vi "HVAC_Control_subTest.vi"(7 "Test Result in":T2=enum."Success", 8 "error in":errorcluster, 9 "DeviceID":T1, 10 "MicrogridID":u8, 11 "Message Enqueuer in":refnum<class "Message Enqueuer.lvclass">) -> (0 "error out":errorcluster, 1 "dup DeviceID":T1, 2 "dup MicrogridID":u8, 3 "Message Enqueuer out":refnum<class "Message Enqueuer.lvclass">, 5 "Test Result out":T2=enum."Success")   [LabVIEW 2018, in "IED Test Framework.lvlib" / "IED Test.lvclass"]
doc: "This VI tests Activate and Deactive messages as part of DER_Control."
uses:
  IED Test.lvclass
  Controls/Test Result.ctl
  <vilib>/ORNL/CSEISMIC DDS/CSEISMIC DDS Base/Data Types/Controls/DeviceID.ctl
  <vilib>/ActorFramework/Message Enqueuer/Message Enqueuer.lvclass
  <vilib>/ORNL/CSEISMIC DDS/CSEISMIC DDS Base/Data Types/Controls/ControlMode.ctl
  <vilib>/ORNL/CSEISMIC DDS/CSEISMIC DDS Base/Data Types/HVAC_Control.ctl
  <vilib>/ORNL/CSEISMIC DDS/CSEISMIC DDS Base/CSEISMIC DDS.lvclass/CSEISMIC DDS.ctl
  HVAC Actor/HVAC Messages/Write HVAC Control Msg/Write HVAC Control Msg.lvclass/Write HVAC Control Msg.ctl
  <vilib>/ActorFramework/Message Enqueuer/Message Enqueuer.lvclass/Message Enqueuer.ctl
  <vilib>/ORNL/CSEISMIC DDS/CSEISMIC DDS Base/Accessors/Write DDS Reference.vi
  <vilib>/ActorFramework/Message Enqueuer/Enqueue.vi
  <vilib>/ORNL/CSEISMIC DDS/CSEISMIC DDS Base/Accessors/Read DDS Reference.vi
  <vilib>/ORNL/CSEISMIC DDS/DDS Reader/DDS Reader.lvclass
  C:/Program Files (x86)/National Instruments/LabVIEW 2018/vi.lib/ORNL/CSEISMIC DDS/CSEISMIC DDS Base/CSEISMIC DDS.lvclass
  HVAC Actor/HVAC Messages/Write HVAC Control Msg/Write HVAC Control Msg.lvclass
  C:/Program Files (x86)/National Instruments/LabVIEW 2018/vi.lib/ActorFramework/Message/Message.lvclass
  <vilib>/ORNL/CSEISMIC DDS/CSEISMIC DDS Base/Error Handler.vi
  <vilib>/ActorFramework/Message Priority Queue/Priority Enqueue.vi
  <vilib>/ORNL/CSEISMIC DDS/CSEISMIC DDS Base/CSEISMIC DDS.lvclass
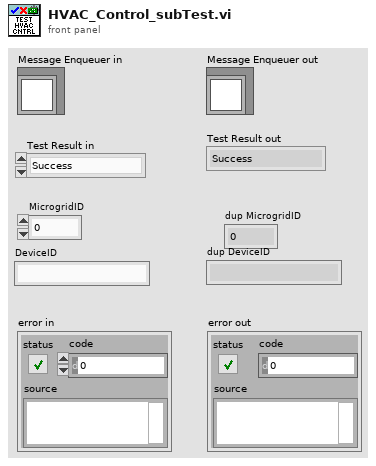
[diagram p1: front panel]
types:
  T1 = typedef "CSEISMIC DDS.lvlib/CSEISMIC DDS.lvclass/DeviceID.ctl" = string
  T2 = typedef "IED Test Framework.lvlib/IED Test.lvclass/Test Result.ctl" = enum16{"Invalid", "Success", "Failure", "Error", "Timeout"}
  T3 = typedef "CSEISMIC DDS.lvlib/CSEISMIC DDS.lvclass/ControlMode.ctl" = enum32{"Invalid", "Cooling", "Heating"}
  T4 = typedef "CSEISMIC DDS.lvlib/CSEISMIC DDS.lvclass/HVAC_Control.ctl" = cluster{"DeviceID":T1, "Temperature(degC)":dbl, "ControlMode":T3}
  T5 = typedef "LVDDS_library.lvlib/DDS Sample Info.ctl" = cluster{"DDS_SampleStateKind":enum32{"DDS_INVALID_SAMPLE_STATE", "DDS_READ_SAMPLE_STATE", "DDS_NOT_READ_SAMPLE_STATE"}, "DDS_ViewStateKind":enum32{"DDS_INVALID_SAMPLE_STATE", "DDS_NEW_VIEW_STATE", "DDS_NOT_NEW_VIEW_STATE"}, "DDS_InstanceStateKind":enum32{"DDS_INVALID_STATE", "DDS_ALIVE_INSTANCE_STATE", "DDS_NOT_ALIVE_DISPOSED_INSTANCE_STATE", "", "DDS_NOT_ALIVE_NO_WRITERS_INSTANCE_STATE"}, "sec":i32, "nanosec":u32, "valid_data":bool}
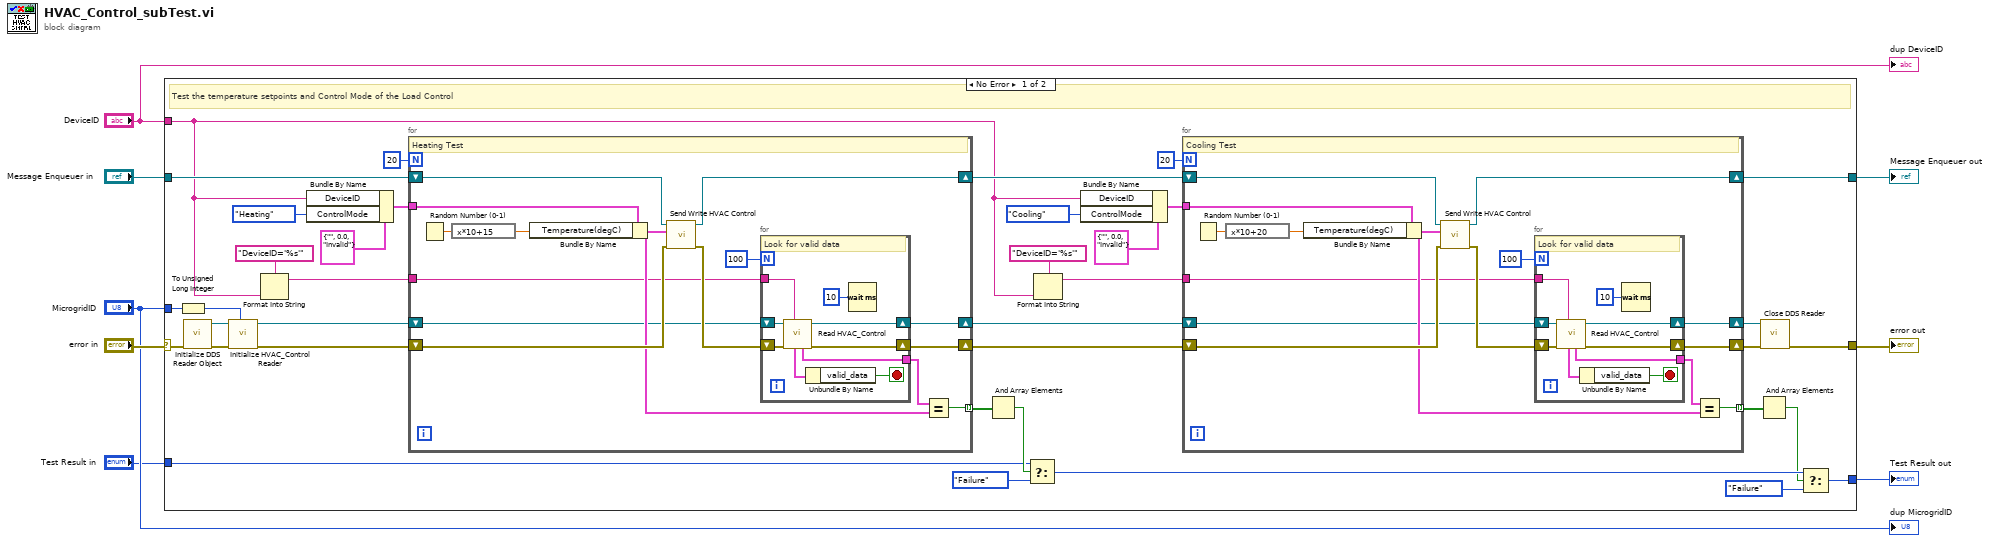
[diagram p0: block diagram]
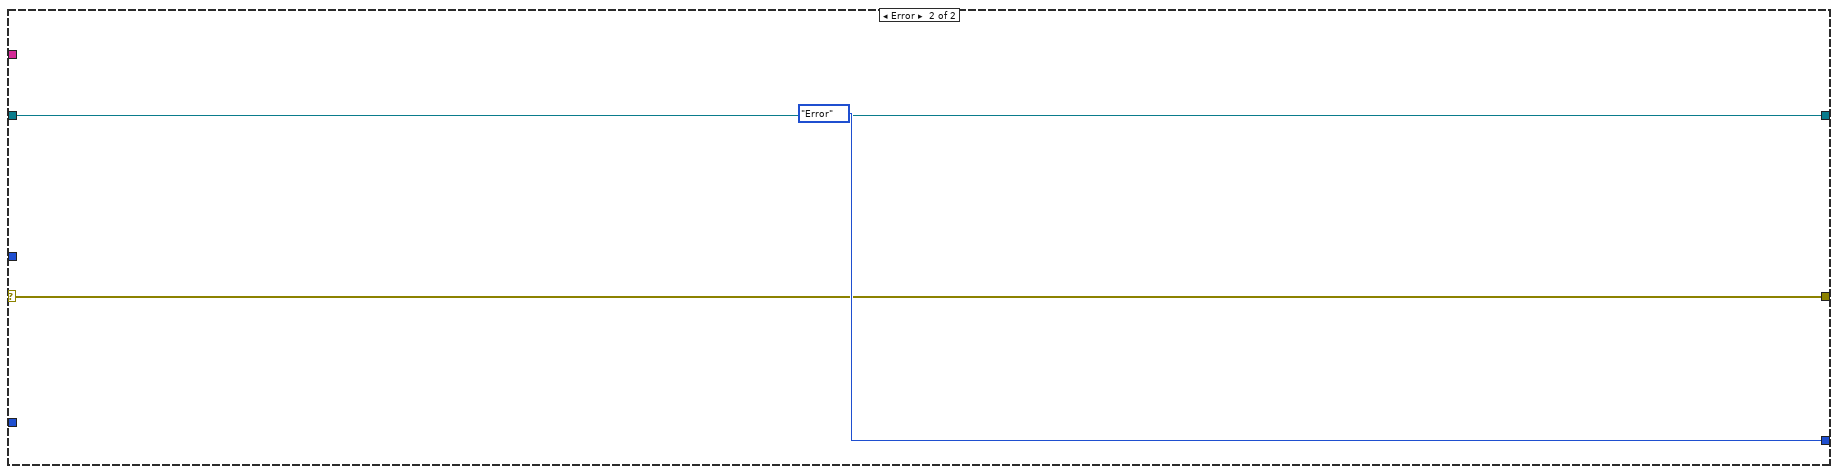
[diagram p2: hidden frame]
diagram:
  n1 = case shown="No Error" "error in" {
    selector: "error in" -> [w33 w95]
    tunnel: [w35 Test_Result."Error" ("Test Result")] -> w8
    tunnel: "DeviceID" -> [w14 _]
    tunnel: [w9 w94] -> w7
    tunnel: "MicrogridID" -> [w32 _]
    tunnel: [w10 w95] -> w6
    tunnel: "Message Enqueuer in" -> [w42 w94]
    tunnel: "Test Result in" -> [w38 _]
    frame No Error {
      # "Test the temperature setpoints and Control Mode of the Load Control"
      n2 = To Unsigned Long Integer(number=w32) -> (unsigned 32bit integer=w29:u32)
      n3 = call <vilib>:"Initialize DDS Reader Object.vi"("error in"=w33) -> ("error out"=w31:errorcluster, "DDS Reader out"=w30:refnum<class "DDS Reader.lvclass">)  [unwired: 9 in]
      n4 = call <vilib>:"Initialize HVAC_Control Reader.vi"("MicrogridID"=w29, "error in"=w31, "DDS Reader in"=w30) -> ("error out"=w28:errorcluster, "DDS Reader out"=w27:refnum<class "DDS Reader.lvclass">)  [unwired: 7 in]
      n5 = Format Into String(format string="DeviceID='%s'", w14) -> (resulting string=w25:string)  [unwired: 2 in, 1 out]
      n6 = Bundle By Name(cluster=T4 {"DeviceID"="", "Temperature(degC)"=0.0, "ControlMode"=enum."Invalid"} ("HVAC_Control"), "DeviceID"=w14, "ControlMode"=ControlMode."Heating") -> (w43:T4)
      n7 = for {
        N: 20 -> [_]
        tunnel: w43 -> [w84]
        shift-right: [w80] -> w17
        shift-left: w42 -> [w81]
        shift-right: [w70] -> w15
        shift-left: w28 -> [w79]
        tunnel: [w76] -> w41 mode=indexing
        shift-right: [w71] -> w16
        shift-left: w27 -> [w73]
        tunnel: w25 -> [w72]
        # "Heating Test"
        n8 = Random Number (0-1)() -> (number: 0 to 1=w83:dbl)
        n9 = expression code="x*10+15"(w83) -> (w82:dbl)
        n10 = Bundle By Name(cluster=w84, "Temperature(degC)"=w82) -> (w78:T4)
        n11 = call "Send Write HVAC Control.vi"("error in (no error)"=w79, "HVAC_Control"=w78, "Message Enqueuer"=w81) -> ("error out"=w74:errorcluster, "Message Enqueuer out"=w80:refnum<class "Message Enqueuer.lvclass">)  [unwired: 7 in]
        n12 = for {
          N: 100 -> [_]
          tunnel: [w87] -> w77
          shift-right: [w86] -> w70
          shift-left: w74 -> [w85]
          shift-right: [w90] -> w71
          shift-left: w73 -> [w91]
          tunnel: w72 -> [w89]
          stop <- w92 stop-if-true
          # "Look for valid data"
          n13 = call <vilib>:"Read HVAC_Control.vi"("Query condition"=w89, "error in"=w85, "DDS Reader in"=w91) -> ("error out"=w86:errorcluster, "DDS Reader out"=w90:refnum<class "DDS Reader.lvclass">, "data"=w87:T4, "DDS Sample Info"=w88:T5)  [unwired: 5 in]
          n14 = Unbundle By Name(w88) -> ("valid_data"=w92:bool)
          n15 = Wait (ms)(milliseconds to wait=u32 10) -> ()  [unwired: 1 out]
        }
        n16 = Equal?(x=w77, y=w78) -> (x = y?=w76:bool)
      }
      n17 = And Array Elements(Boolean array=w41) -> (logical AND=w39:bool)
      n18 = Select(t=w38, s=w39, f=Test_Result."Failure" ("Test Result")) -> (s? t:f=w36:T2)
      n19 = Format Into String(format string="DeviceID='%s'", w14) -> (resulting string=w24:string)  [unwired: 2 in, 1 out]
      n20 = Bundle By Name(cluster=T4 {"DeviceID"="", "Temperature(degC)"=0.0, "ControlMode"=enum."Invalid"} ("HVAC_Control"), "DeviceID"=w14, "ControlMode"=ControlMode."Cooling") -> (w20:T4)
      n21 = for {
        N: 20 -> [_]
        tunnel: w20 -> [w60]
        shift-right: [w56] -> w9
        shift-left: w17 -> [w57]
        shift-right: [w46] -> w11
        shift-left: w15 -> [w55]
        tunnel: [w52] -> w21 mode=indexing
        shift-right: [w47] -> w12
        shift-left: w16 -> [w49]
        tunnel: w24 -> [w48]
        # "Cooling Test"
        n22 = Random Number (0-1)() -> (number: 0 to 1=w59:dbl)
        n23 = expression code="x*10+20"(w59) -> (w58:dbl)
        n24 = Bundle By Name(cluster=w60, "Temperature(degC)"=w58) -> (w54:T4)
        n25 = call "Send Write HVAC Control.vi"("error in (no error)"=w55, "HVAC_Control"=w54, "Message Enqueuer"=w57) -> ("error out"=w50:errorcluster, "Message Enqueuer out"=w56:refnum<class "Message Enqueuer.lvclass">)  [unwired: 7 in]
        n26 = for {
          N: 100 -> [_]
          tunnel: [w63] -> w53
          shift-right: [w62] -> w46
          shift-left: w50 -> [w61]
          shift-right: [w66] -> w47
          shift-left: w49 -> [w67]
          tunnel: w48 -> [w65]
          stop <- w68 stop-if-true
          # "Look for valid data"
          n27 = call <vilib>:"Read HVAC_Control.vi"("Query condition"=w65, "error in"=w61, "DDS Reader in"=w67) -> ("error out"=w62:errorcluster, "DDS Reader out"=w66:refnum<class "DDS Reader.lvclass">, "data"=w63:T4, "DDS Sample Info"=w64:T5)  [unwired: 5 in]
          n28 = Unbundle By Name(w64) -> ("valid_data"=w68:bool)
          n29 = Wait (ms)(milliseconds to wait=u32 10) -> ()  [unwired: 1 out]
        }
        n30 = Equal?(x=w53, y=w54) -> (x = y?=w52:bool)
      }
      n31 = And Array Elements(Boolean array=w21) -> (logical AND=w13:bool)
      n32 = call <vilib>:"Close DDS Reader.vi"("error in"=w11, "DDS Reader in"=w12) -> ("error out"=w10:errorcluster)  [unwired: 9 in]
      n33 = Select(t=w36, s=w13, f=Test_Result."Failure" ("Test Result")) -> (s? t:f=w35:T2)
    }
    frame Error {
    }
  }
  "Test Result out" <- w8
  "Message Enqueuer out" <- w7
  "error out" <- w6
  "dup MicrogridID" <- "MicrogridID"
  "dup DeviceID" <- "DeviceID"
